vi "PH_Calorimeter_USB.PC Write PSDB.vi"(0 "i ref in":refnum<vi>, 5 "error IO":errorcluster) -> (14 "i ref out":refnum<vi>, 19 "error out":errorcluster)   [LabVIEW 2014, in "PH_Calorimeter_USB.lvlib"]
doc: "This is the proc case which writes data to the PHELIX shot data base."
uses:
  PH_Calorimeter_USB.lvlib
  PH_Basics/PH_PSDBWriter/PH_PSDBWriter.2D dataset.ctl
  CSlibraries-extern/psdb_lv/PSDB_AxisDescription.ctl
  PH_Basics/PH_Common/PH_Common.lvlib
  PH_Basics/PH_PSDBWriter/PH_PSDBWriter.lvlib
  CSlibraries-extern/psdb_lv/PSDB.lvlib
panel:
  in  "axis description":T1
  in  "2D data":T2
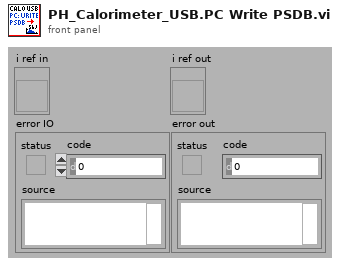
[diagram p1: front panel]
types:
  T1 = typedef "PSDB.lvlib/PSDB_AxisDescription.ctl" = cluster{"x axis label":string, "y axis label":string, "x axis unit":string, "y axis unit":string}
  T2 = typedef "PH_PSDBWriter.lvlib/PH_PSDBWriter.2D dataset.ctl" = cluster{"name":string, "data":dbl[][], "axis description":T1}
  T3 = typedef "PH_Calorimeter_USB.lvlib/PH_Calorimeter_USB.i attribute.ctl" = cluster{"GUI Refs":cluster{"Delete":refnum<vi>, "Start":refnum<vi>, "Energy":refnum<vi>, "Calorimeter":refnum<vi>, "Trigger":refnum<vi>, "Calo Calibration":refnum<vi>, "Time Base":refnum<vi>, "Device":refnum<vi>, "Graph Raw Data":refnum<vi>, "Graph Result":refnum<vi>}, "DAQ Instance":string, "Data":dbl[][], "Controller Instance":string, "Energy [J]":dbl, "Calorimeter":T4, "Trigger":T5, "Time Base":T6, "Calo Calibration":T7, "Serial Number":string}
  T4 = typedef "PH_Calorimeter_USB.lvlib/PH_Calorimeter_USB.Calorimeter Settings.ctl" = cluster{"Channel":tag, "Min Value [V]":dbl, "Max Value  [V]":dbl}
  T5 = typedef "PH_Calorimeter_USB.lvlib/PH_Calorimeter_USB.Trigger Settings.ctl" = cluster{"Channel":tag, "Min Value [V]":dbl, "Max Value  [V]":dbl, "Level [V]":dbl, "Wait Time [s]":dbl, "Length [Samples]":i32}
  T6 = typedef "PH_Calorimeter_USB.lvlib/PH_Calorimeter_USB.Time Base Settings.ctl" = cluster{"Samples per Channel":i32, "Rate [Hz]":i32}
  T7 = typedef "PH_Calorimeter_USB.lvlib/PH_Calorimeter_USB.Calorimeter Calibration Settings.ctl" = cluster{"T 1/e [s]":dbl, "Sensitivity  [Vs/J]":dbl}
  T8 = typedef "PH_PSDBWriter.lvlib/PH_PSDBWriter.Numeric dataset.ctl" = cluster{"name":string, "data":dbl, "unit":string}
  T9 = typedef "PH_PSDBWriter.lvlib/PH_PSDBWriter.String dataset.ctl" = cluster{"name":string, "data":string, "unit":string}
  T10 = typedef "PH_PSDBWriter.lvlib/PH_PSDBWriter.PSDB Dataset.ctl" = cluster{"Version":i32, "2D data Input":T2[], "Boolean Input":T11[], "Image Input":T12[], "Numeric Input":T8[], "String Input":T9[]}
  T11 = typedef "PH_PSDBWriter.lvlib/PH_PSDBWriter.Boolean dataset.ctl" = cluster{"name":string, "data":bool, "unit":string}
  T12 = typedef "PH_PSDBWriter.lvlib/PH_PSDBWriter.Image dataset.ctl" = cluster{"name":string, "data":T13, "unit":string}
  T13 = typedef "IMAQ Image.ctl" = refnum<image>
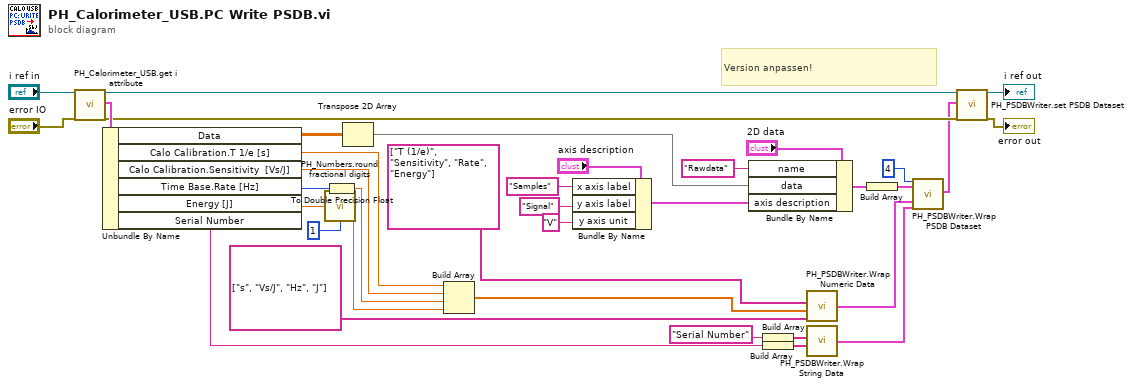
[diagram p0: block diagram]
diagram:
  # "Version anpassen!"
  n1 = call "PH_Calorimeter_USB.get i attribute.vi"("i ref in"="i ref in", "error in (no error)"="error IO") -> ("i ref out"=w14:refnum<vi>, "i attribute"=w34:T3, "error out"=w33:errorcluster)  [unwired: 15 in]
  n2 = Unbundle By Name(w34) -> ("Data"=w30:dbl[][], "Calo Calibration.T 1/e [s]"=w19:dbl, "Calo Calibration.Sensitivity  [Vs/J]"=w20:dbl, "Time Base.Rate [Hz]"=w23:i32, "Energy [J]"=w21:dbl, "Serial Number"=w9:string)
  n3 = call "PH_Numbers.round fractional digits.vi"("Input"=w21, "Position (1)"=i16 1) -> ("round Output"=w18:dbl)
  n4 = To Double Precision Float(number=w23) -> (double precision float=w22:dbl)
  n5 = Transpose 2D Array(2D array=w30) -> (transposed array=w16:dbl[][])
  n6 = Build Array(w19, w20, w22, w18) -> (w3:dbl[])
  n7 = Bundle By Name(cluster="axis description", "x axis label"="Samples", "y axis label"="Signal", "y axis unit"="V") -> (w27:T1)
  n8 = Bundle By Name(cluster="2D data", "name"="Rawdata", "data"=w16, "axis description"=w27) -> (w29:T2)
  n9 = Build Array("Serial Number" ("name")) -> (w5:string[])
  n10 = Build Array(w9) -> (w6:string[])
  n11 = call "PH_PSDBWriter.Wrap Numeric Data.vi"("Unit Array"=string[] ["s", "Vs/J", "Hz", "J"], "Data Array"=w3, "Name Array"=string[] ["T (1/e)", "Sensitivity", "Rate", "Energy"]) -> ("PSDB Numeric Data Array"=w1:T8[])  [unwired: 1 in]
  n12 = call "PH_PSDBWriter.Wrap String Data.vi"("Data Array"=w6, "Name Array"=w5) -> ("PSDB String Data Array"=w7:T9[])  [unwired: 2 in]
  n13 = Build Array(w29) -> (w11:T2[])
  n14 = call "PH_PSDBWriter.Wrap PSDB Dataset.vi"("Version"=4, "2D data Input"=w11, "Numeric Input"=w1, "String Input"=w7) -> ("PSDB Dataset"=w10:T10)  [unwired: 15 in]
  n15 = call "PH_PSDBWriter.set PSDB Dataset.vi"("VI in"=w14, "PSDB Dataset"=w10, "error in (no error)"=w33) -> ("VI out"=→"i ref out":refnum<vi>, "error out"=→"error out":errorcluster)  [unwired: 15 in]
